vi "ReadEXCEL_210928.vi"(8 "错误输入（无错误）":errorcluster, 9 "EXCEL 标签":string="Sheet1", 10 "路径":path, 11 "自动化引用句柄":refnum<k7>) -> (0 "错误输出":errorcluster, 1 "数据":string[][](array[string]))   [LabVIEW 2018]
panel:
  in  "数组":string[][](array[string])
  in  "Excel._Worksheet":refnum<k7>
  in  "Excel._Application":refnum<k7>
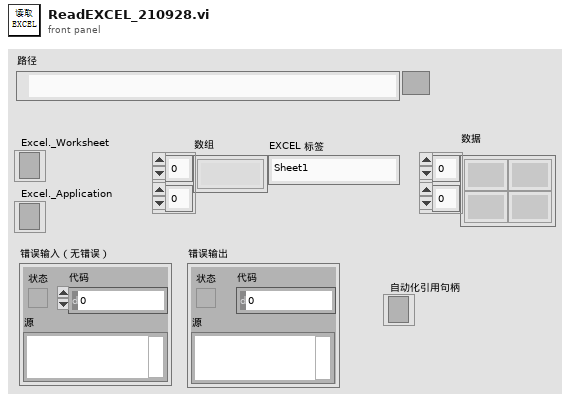
[diagram p1: front panel]
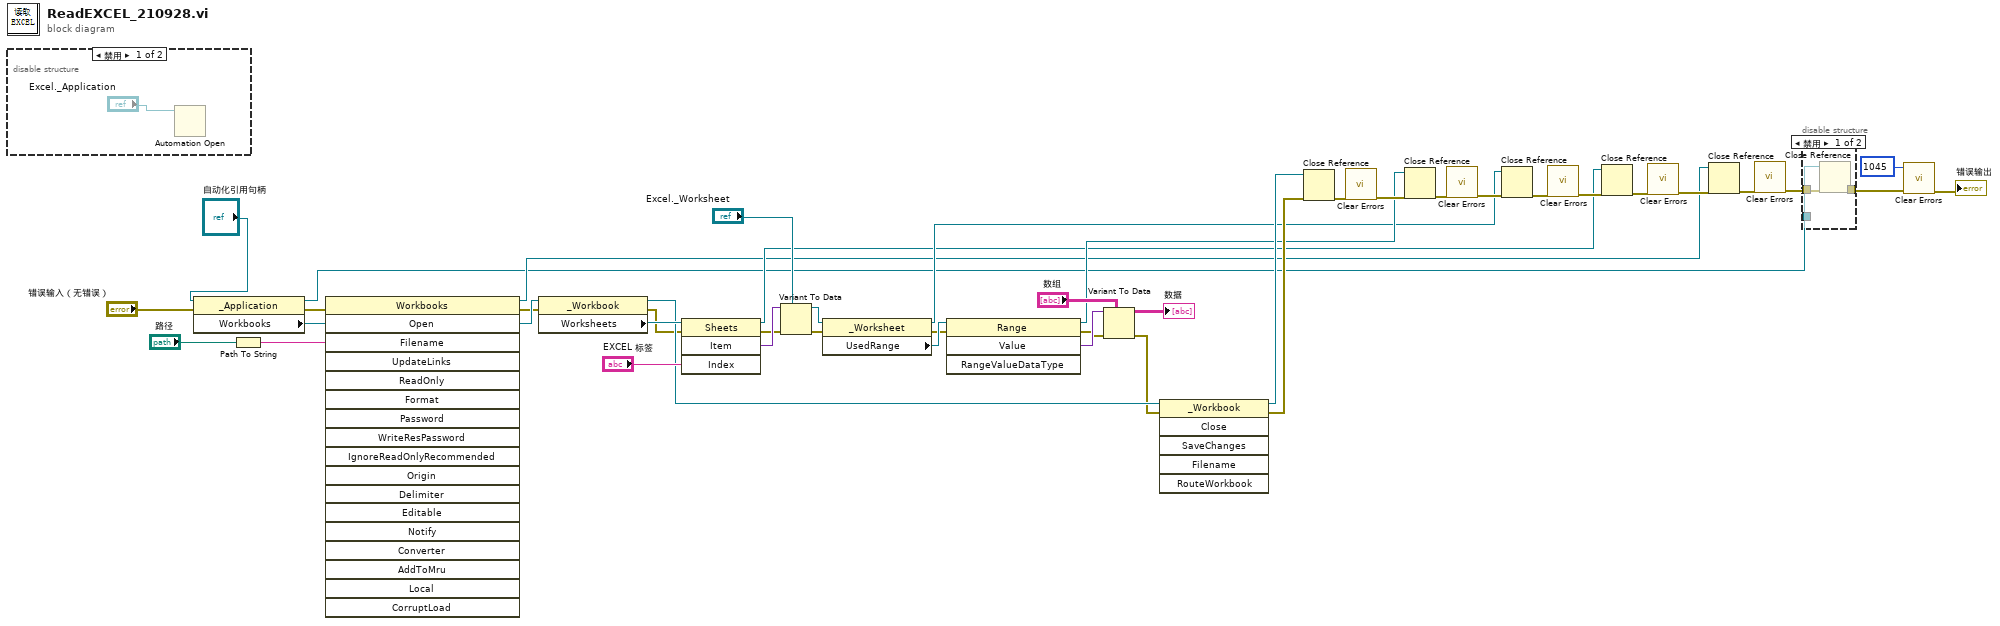
[diagram p0: block diagram]
diagram:
  n1 = disable-structure shown="禁用" {
    frame Disabled {
      n2 = Automation Open(Automation Refnum="Excel._Application") -> ()  [unwired: 1 in, 4 out]
    }
    frame Enabled {
    }
  }
  n3 = property class="_Application"(reference="自动化引用句柄", error in="错误输入（无错误）") -> (reference out=w6:refnum<k7>, error out=w44:errorcluster, "Workbooks"=w29:refnum<k7>)
  n4 = Path To String(path="路径") -> (string=w28:string)
  n5 = invoke class="Workbooks" method="Open"(reference=w29, error in=w44, "Filename"=w28) -> (reference out=w8:refnum<k7>, error out=w42:errorcluster, "Open"=w43:refnum<k7>)  [unwired: 15 in, 15 out]
  n6 = property class="_Workbook"(reference=w43, error in=w42) -> (reference out=w27:refnum<k7>, error out=w23:errorcluster, "Worksheets"=w41:refnum<k7>)
  n7 = invoke class="Sheets" method="Item"(reference=w41, error in=w23, "Index"="EXCEL 标签") -> (reference out=w11:refnum<k7>, error out=w38:errorcluster, "Item"=w40:variant)  [unwired: 1 in, 1 out]
  n8 = Variant To Data(error in=w38, type="Excel._Worksheet", Variant=w40) -> (data=w37:refnum<k7>, error out=w34:errorcluster)
  n9 = property class="_Worksheet"(reference=w37, error in=w34) -> (reference out=w14:refnum<k7>, error out=w33:errorcluster, "UsedRange"=w36:refnum<k7>)
  n10 = invoke class="Range" method="Value"(reference=w36, error in=w33) -> (reference out=w15:refnum<k7>, error out=w32:errorcluster, "Value"=w35:variant)  [unwired: 2 in, 1 out]
  n11 = Variant To Data(error in=w32, type="数组", Variant=w35) -> (data=→"数据":string[][], error out=w26:errorcluster)
  n12 = invoke class="_Workbook" method="Close"(reference=w27, error in=w26) -> (reference out=w16:refnum<k7>, error out=w21:errorcluster)  [unwired: 4 in, 4 out]
  n13 = Close Reference(reference=w16, error in (no error)=w21) -> (error out=w22:errorcluster)
  n14 = call <vilib>:"Clear Errors.vi"("error in (no error)"=w22) -> ("error out"=w18:errorcluster)  [unwired: 5 in, 1 out]
  n15 = Close Reference(reference=w15, error in (no error)=w18) -> (error out=w20:errorcluster)
  n16 = call <vilib>:"Clear Errors.vi"("error in (no error)"=w20) -> ("error out"=w17:errorcluster)  [unwired: 5 in, 1 out]
  n17 = Close Reference(reference=w14, error in (no error)=w17) -> (error out=w19:errorcluster)
  n18 = call <vilib>:"Clear Errors.vi"("error in (no error)"=w19) -> ("error out"=w12:errorcluster)  [unwired: 5 in, 1 out]
  n19 = Close Reference(reference=w11, error in (no error)=w12) -> (error out=w13:errorcluster)
  n20 = call <vilib>:"Clear Errors.vi"("error in (no error)"=w13) -> ("error out"=w9:errorcluster)  [unwired: 5 in, 1 out]
  n21 = Close Reference(reference=w8, error in (no error)=w9) -> (error out=w10:errorcluster)
  n22 = call <vilib>:"Clear Errors.vi"("error in (no error)"=w10) -> ("error out"=w7:errorcluster)  [unwired: 5 in, 1 out]
  n23 = disable-structure shown="禁用" {
    disable-tunnel: w7 -> [w48 _]
    disable-tunnel: w6 -> [w47 _]
    disable-tunnel: [w46 _] -> w5
    frame Disabled {
      n24 = Close Reference(reference=w47, error in (no error)=w48) -> (error out=w46:errorcluster)
    }
    frame Enabled {
    }
  }
  n25 = call <vilib>:"Clear Errors.vi"("error in (no error)"=w5, "specific error code to clear (0: all)"=1045) -> ("error out"=→"错误输出":errorcluster)  [unwired: 4 in, 1 out]
